vi "Interepter.vi"(11 "Array":string[][](array[string])) -> ()   [LabVIEW 2011]
uses:
  <vilib>/regexp/Match Regular Expression.xnode
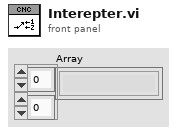
[diagram p1: front panel]
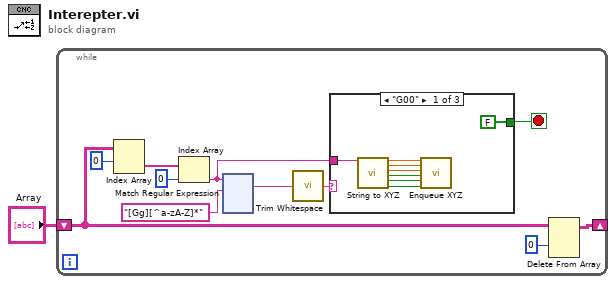
[diagram p0: block diagram]
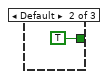
[diagram p2: hidden frame]
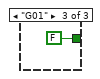
[diagram p3: hidden frame]
diagram:
  n1 = while {
    shift-right: [w11] -> _
    shift-left: "Array" -> [w8]
    stop <- w9 stop-if-true
    n2 = Index Array(array=w8, index (row)=0) -> (element=w7:string[])  [unwired: 1 in]
    n3 = Index Array(array=w7, index=0 ("index (row)")) -> (element=w3:string)
    n4 = xnode "Match Regular Expression"("input string"=w3, "regular expression"="[Gg][^a-zA-Z]*") -> ("whole match"=w4:string)  [unwired: 4 in, 4 out]
    n5 = call <vilib>:"Trim Whitespace.vi"("string"=w4) -> ("trimmed string"=w2:string)  [unwired: 1 in]
    n6 = case shown="\"G00\"" w2 {
      tunnel: [FALSE TRUE FALSE] -> w9
      tunnel: w3 -> [w130 _ _]
      frame "G00" {
        n7 = call "String to XYZ.vi"("Input string"=w130) -> ("X"=w129:dbl, "Y"=w128:dbl, "Z"=w127:dbl, "X Has Value?"=w126:bool, "Y Has Value?"=w125:bool, "Z Has Value?"=w124:bool)  [unwired: 13 in]
        n8 = call "Enqueue XYZ.vi"("X"=w129, "Y"=w128, "Z"=w127, "X Has Value?"=w126, "Y Has Value?"=w125, "Z Has Value?"=w124) -> ()  [unwired: 14 in]
      }
      frame Default {
      }
      frame "G01" {
      }
    }
    n9 = Delete From Array(array=w8, index (row)=0) -> (array with subset deleted=w11:string[][])  [unwired: 2 in, 1 out]
  }
